vi "Read Int.vi"(8 "error in (no error)":errorcluster, 11 "VISA resource name In":refnum<visa-resource-name>) -> (0 "error out":errorcluster, 2 "int":u32, 3 "VISA resource name out":refnum<visa-resource-name>)   [LabVIEW 2009, in "Newport 1830-C.lvlib"]
doc: "Reads the and unsigned 32-bit integer from the output buffer of the instrument."
uses:
  Newport 1830-C.lvlib
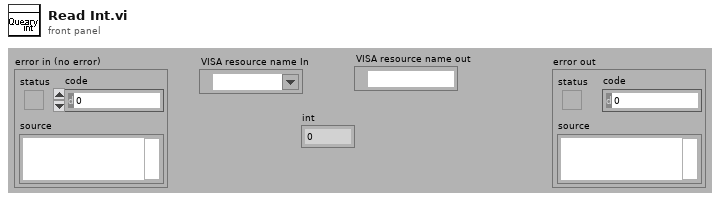
[diagram p1: front panel]
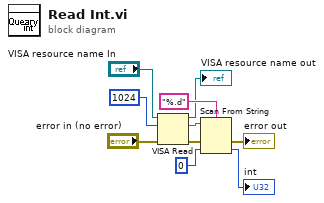
[diagram p0: block diagram]
diagram:
  n1 = VISA Read(VISA resource name="VISA resource name In", byte count=u32 1024, error in (no error)="error in (no error)") -> (VISA resource name out=→"VISA resource name out":refnum<visa-resource-name>, read buffer=w9:string, error out=w8:errorcluster)  [unwired: 1 out]
  n2 = Scan From String(format string="%.d", input string=w9, error in=w8, default 1=u32 0) -> (error out=→"error out":errorcluster, output 1=→"int":u32)  [unwired: 1 in, 2 out]
